vi "file(read from text).vi"() -> ()   [LabVIEW 2020]
panel:
  out "all upper case string":string
  out "length":i32
  in  "file path (use dialog)":path
  out "text":string
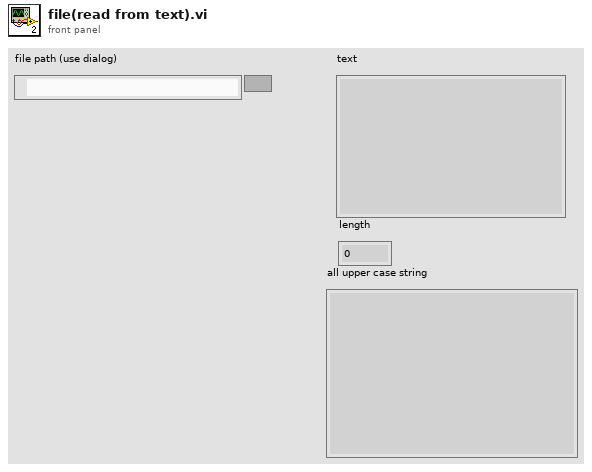
[diagram p1: front panel]
types:
  T1 = enum16{"open", "replace", "create", "open or create", "replace or create", "replace or create with confirmation"}
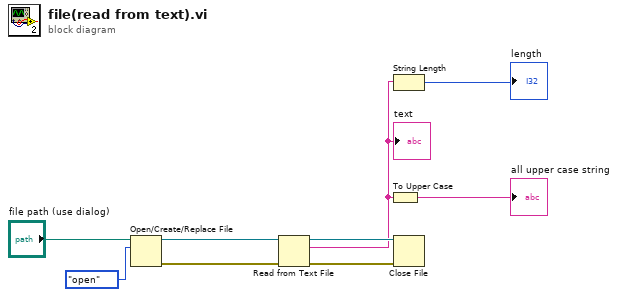
[diagram p0: block diagram]
diagram:
  n1 = Open/Create/Replace File(file path (use dialog)="file path (use dialog)", operation (0:open)=T1."open") -> (refnum out=w9:refnum<file>, error out=w7:errorcluster)  [unwired: 4 in, 1 out]
  n2 = Read from Text File(file (use dialog)=w9, error in=w7) -> (refnum out=w8:refnum<file>, text=w2:string, error out=w6:errorcluster)  [unwired: 2 in, 1 out]
  "text" <- w2
  n3 = To Upper Case(1:w2) -> (0:→"all upper case string":string)
  n4 = String Length(string=w2) -> (length=→"length":i32)
  n5 = Close File(refnum=w8, error in=w6) -> ()  [unwired: 2 out]
